vi "Create triangles mesh.vi"(2 "Colour":T2={"Red"=1.0, "Green"=1.0, "Blue"=1.0, "Alpha"=1.0}, 3 "Render mode":T3(ring)=enum."Polygons", 4 "Triangles array":T1[](array[typedef])) -> (0 "Error out":errorcluster, 1 "Triangle mesh out":refnum<vi>)   [LabVIEW 2022 SP3]
uses:
  <vilib>/Utility/miscctls.llb/LVRGBAColorTypeDef.ctl
  Typedefs/Triangle.ctl
  <vilib>/Utility/miscctls.llb/LV3DPointTypeDef.ctl
  <vilib>/picture/3D Picture Control/Object/Create Object (drawable).vi
  <vilib>/picture/3D Picture Control/NI_3D Picture Control.lvlib
panel:
  in  "Shininess":sgl=128.0 min=0 max=128
  out "ambient":u32(colorbox)
  out "diffuse":u32(colorbox)
  # "PN 19/01/2015"
  # "Vertices"
  # "Edges"
  # "Unit normal"
  # "Edge unit normals"
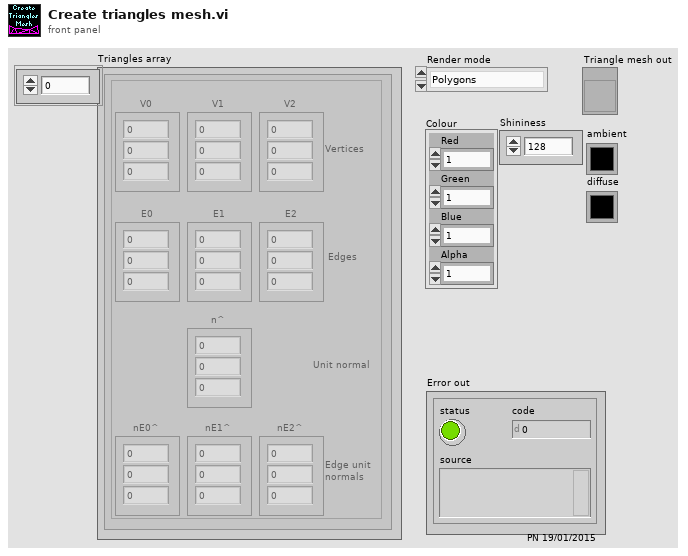
[diagram p1: front panel]
types:
  T1 = typedef "Triangle.ctl" = cluster{"V0":sgl[], "V1":sgl[], "V2":sgl[], "E0":sgl[], "E1":sgl[], "E2":sgl[], "n^":sgl[], "nE0^":sgl[], "nE1^":sgl[], "nE2^":sgl[]}
  T2 = typedef "LVRGBAColorTypeDef.ctl" = cluster{"Red":sgl, "Green":sgl, "Blue":sgl, "Alpha":sgl}
  T3 = enum16{"Inherit Value", "Points", "Wireframe", "Polygons"}
  T4 = enum16{"Overall", "Per Primitive", "Per Vertex", "Binding Off"}
  T5 = enum16{"Points", "Lines", "Line Strip", "Line Loop", "Triangles", "Triangle Strip", "Triangle Fan", "Quads", "Quad Strip", "Polygon"}
  T6 = enum16{"Inherit Value", "No Culling", "Cull Back Face", "Cull Front Face", "Cull Both Faces"}
  T7 = enum16{"Inherit Value", "Counterclockwise", "Clockwise"}
  T8 = typedef "LV3DPointTypeDef.ctl" = cluster{"X":sgl, "Y":sgl, "Z":sgl}
  T9 = enum16{"Inherit Material", "Use entire Material", "Ignore Ambient", "Ignore Diffuse", "Ignore Specular", "Ignore Emission", "Ignore Ambient and Diffuse"}
  T10 = enum16{"Normal Bin", "Opaque Bin", "Transparent Bin"}
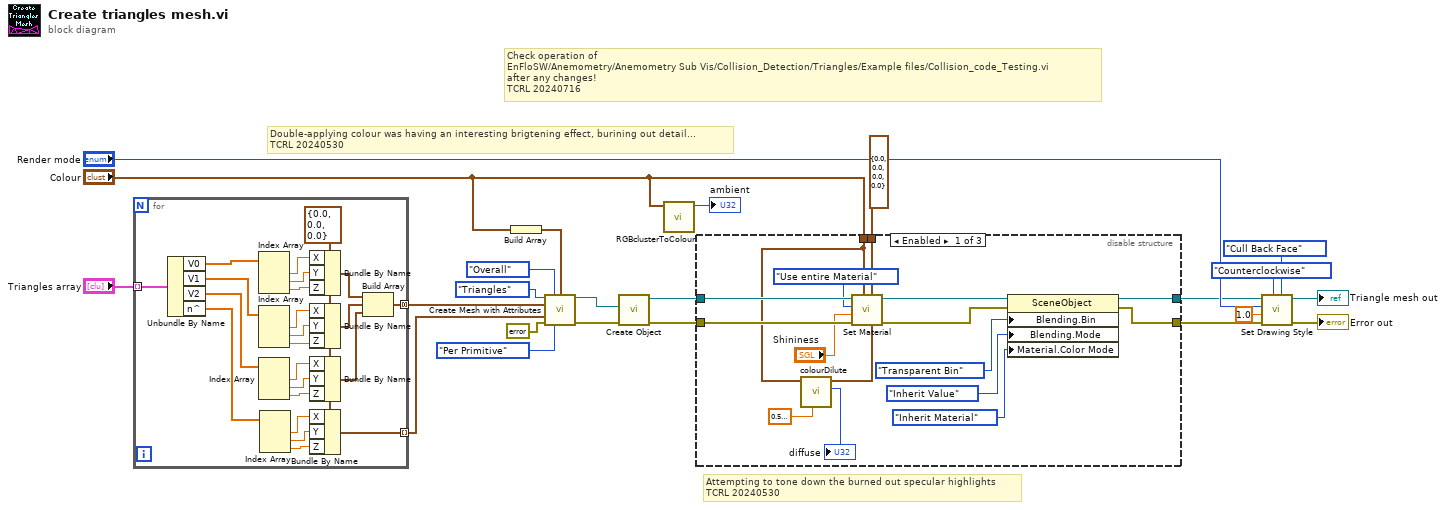
[diagram p0: block diagram]
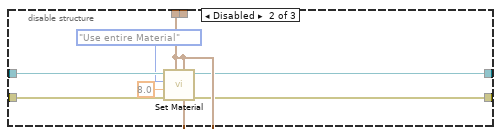
[diagram p2: hidden frame]
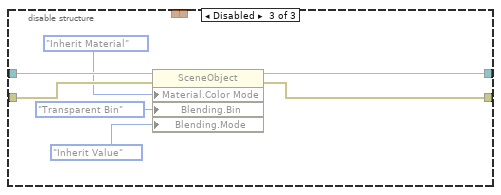
[diagram p3: hidden frame]
diagram:
  # "Check operation of\nEnFloSW/Anemometry/Anemometry Sub Vis/Collision_Detection/Triangles/Example files/Collision_code_Testing.vi\nafter any changes!\nTCRL 20240716"
  # "Attempting to tone down the burned out specular highlights\nTCRL 20240530"
  # "Double-applying colour was having an interesting brigtening effect, burining out detail...\nTCRL 20240530"
  n1 = for {
    tunnel: "Triangles array" -> [w46] mode=indexing
    tunnel: [w30] -> w15 mode=concatenating
    tunnel: [w25] -> w14 mode=indexing
    w24 = T8 {"X"=0.0, "Y"=0.0, "Z"=0.0} ("3D Point")
    n2 = Unbundle By Name(w46) -> ("V0"=w45:sgl[], "V1"=w44:sgl[], "V2"=w43:sgl[], "n^"=w27:sgl[])
    n3 = Index Array(array=w45) -> (element #1=w42:sgl, element #2=w40:sgl, element #3=w41:sgl)  [unwired: 3 in]
    n4 = Index Array(array=w44) -> (element #1=w39:sgl, element #2=w38:sgl, element #3=w37:sgl)  [unwired: 3 in]
    n5 = Index Array(array=w43) -> (element #1=w36:sgl, element #2=w35:sgl, element #3=w34:sgl)  [unwired: 3 in]
    n6 = Index Array(array=w27) -> (element #1=w26:sgl, element #2=w28:sgl, element #3=w29:sgl)  [unwired: 3 in]
    n7 = Bundle By Name(cluster=w24, "X"=w42, "Y"=w40, "Z"=w41) -> (w33:T8)
    n8 = Bundle By Name(cluster=w24, "X"=w39, "Y"=w38, "Z"=w37) -> (w32:T8)
    n9 = Bundle By Name(cluster=w24, "X"=w36, "Y"=w35, "Z"=w34) -> (w31:T8)
    n10 = Bundle By Name(cluster=w24, "X"=w26, "Y"=w28, "Z"=w29) -> (w25:T8)
    n11 = Build Array(w33, w32, w31) -> (w30:T8[])
  }
  n12 = Build Array("Colour") -> (w1:T2[])
  n13 = call <vilib>:"Create Mesh with Attributes.vi"("Draw Mode"=T5."Triangles", "Color Binding Mode"=T4."Overall", "Color Array"=w1, "Vertex Array"=w15, "Normal Array"=w14, "error in (no error)"=errorcluster {"status"=FALSE, "code"=0, "source"=""}, "Normal Binding Mode"=T4."Per Primitive") -> ("New Mesh Refnum"=w17:refnum<vi>, "error out"=w18:errorcluster)  [unwired: 7 in]
  n14 = call-poly <vilib>:"Create Object.vi"("error in (no error)"=w18, "Geometry"=w17) -> ("error out"=w6:errorcluster, "Scene:New Object"=w8:refnum<vi>)  [unwired: 8 in]
  n15 = call "RGBclusterToColour.vi"("RGBin"="Colour") -> ("colour"=→"ambient":u32)  [unwired: 10 in]
  n16 = disable-structure shown="Enabled" {
    disable-tunnel: w8 -> [w62 w69 w76]
    disable-tunnel: [w53 w64 w75] -> w7
    disable-tunnel: w6 -> [w60 w68 w74]
    disable-tunnel: [w51 w63 w73] -> w5
    disable-tunnel: "Colour" -> [w54 w65 _]
    disable-tunnel: T2 {"Red"=0.0, "Green"=0.0, "Blue"=0.0, "Alpha"=0.0} ("Specular") -> [w47 _ _]
    frame Enabled {
      n17 = call "colourDilute.vi"("dilutionFactor"=0.5000000000000001, "RGBIn"=w54) -> ("colourOut"=→"diffuse":u32, "RGBOut"=w57:cluster{"R":dbl, "G":dbl, "B":dbl, "A":dbl})  [unwired: 8 in]
      n18 = call <vilib>:"Set Material.vi"("Diffuse"=w57, "Specular"=w47, "Ambient"=w54, "error in (no error)"=w60, "Shininess"="Shininess", "Color Mode"=T9."Use entire Material", "Scene Object In"=w62) -> ("error out"=w52:errorcluster, "Scene Object Out"=w61:refnum<vi>)  [unwired: 3 in]
      n19 = property class="SceneObject"(reference=w61, error in=w52, "Blending.Bin"=T10."Transparent Bin" ("Blending:Bin"), "Blending.Mode"=enum16{"Inherit Value", "Off", "On"}."Inherit Value" ("Blending:Mode"), "Material.Color Mode"=T9."Inherit Material" ("Material:Color Mode")) -> (reference out=w53:refnum<vi>, error out=w51:errorcluster)
    }
    frame Disabled {
      n20 = call <vilib>:"Set Material.vi"("Diffuse"=w65, "Specular"=w65, "Ambient"=w65, "error in (no error)"=w68, "Shininess"=sgl 8.0, "Color Mode"=T9."Use entire Material", "Scene Object In"=w69) -> ("error out"=w63:errorcluster, "Scene Object Out"=w64:refnum<vi>)  [unwired: 3 in]
    }
    frame Disabled {
      n21 = property class="SceneObject"(reference=w76, error in=w74, "Material.Color Mode"=T9."Inherit Material" ("Material:Color Mode"), "Blending.Bin"=T10."Transparent Bin" ("Blending:Bin"), "Blending.Mode"=enum16{"Inherit Value", "Off", "On"}."Inherit Value" ("Blending:Mode")) -> (reference out=w75:refnum<vi>, error out=w73:errorcluster)
    }
  }
  n22 = call <vilib>:"Set Drawing Style.vi"("Face Culling Mode"=T6."Cull Back Face", "Frontface Mode"=T7."Counterclockwise", "error in (no error)"=w5, "Size"=1.0, "Mode"="Render mode", "Scene Object In"=w7) -> ("error out"=→"Error out":errorcluster, "Scene Object Out"=→"Triangle mesh out":refnum<vi>)  [unwired: 4 in]
